vi "provide_OME_data.vi"(6 "image ID":string, 8 "error in (no error)":errorcluster, 9 "structuredAttribute string in":string, 10 "OME element in":refnum<class "XMLElement.lvclass">, 11 "DataCollectionDL091104Scaffold in":refnum<class "DataCollectionDL091104Scaffold.lvclass">) -> (0 "error out":errorcluster, 1 "structuredAttribute string out":string, 2 "OME element out":refnum<class "XMLElement.lvclass">, 3 "DataCollectionDL091104Scaffold out":refnum<class "DataCollectionDL091104Scaffold.lvclass">)   [LabVIEW 2010, in "DataCollectionDL091104Scaffold.lvclass"]
uses:
  DataCollectionDL091104Scaffold.lvclass
  common/classes/XMLElement/XMLElement/XMLElement.lvclass
  GenericDataCollection/GenericDataCollection/GenericDataCollection.lvclass
  DataCollectionDL091104Scaffold.lvclass/DataCollectionDL091104Scaffold.ctl
  Instrument/GenericInstrument/GenericInstrument/GenericInstrument.lvclass
  Objective/GenericObjective/GenericObjective/GenericObjective.lvclass
  common/classes/ErrorController/ErrorController/class_data.vi
  common/classes/ErrorController/ErrorController/ErrorController.lvclass
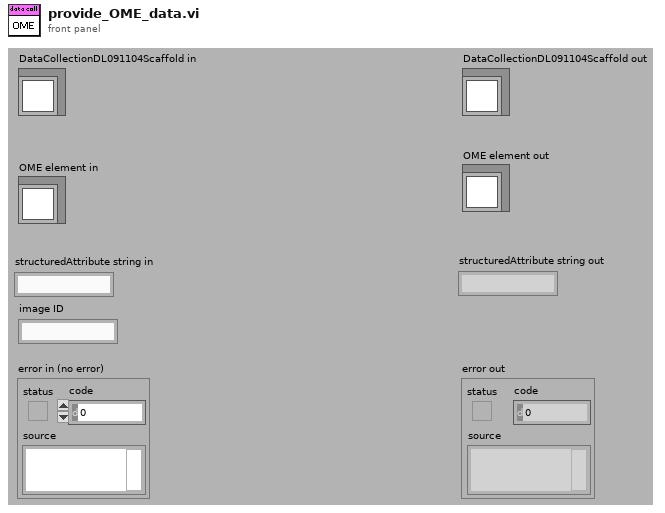
[diagram p1: front panel]
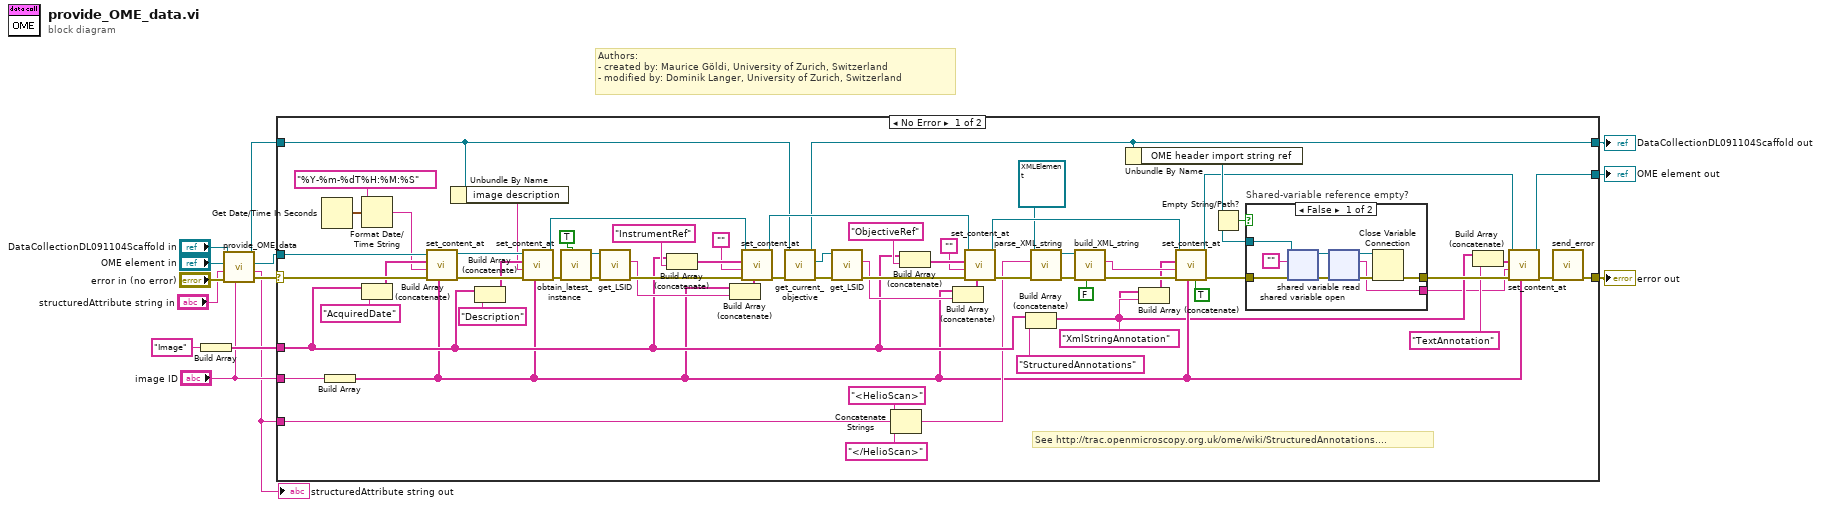
[diagram p0: block diagram]
diagram:
  # "Authors: \n- created by: Maurice Göldi, University of Zurich, Switzerland\n- modified by: Dominik Langer, University of Zurich, Switzerland"
  n1 = Build Array("Image") -> (w10:string[])
  n2 = call-parent "provide_OME_data.vi"("image ID"="image ID", "error in (no error)"="error in (no error)", "structuredAttribute string in"="structuredAttribute string in", "OME element in"="OME element in", "GenericDataCollection in"="DataCollectionDL091104Scaffold in") -> ("error out"=w9:errorcluster, "structuredAttribute string out"=w1:string, "OME element out"=w8:refnum<class "XMLElement.lvclass">, "GenericDataCollection out"=w7:refnum<class "DataCollectionDL091104Scaffold.lvclass">)  [unwired: 3 in]
  "structuredAttribute string out" <- w1
  n3 = case shown="No Error" w9 {
    selector: w9 -> [w71 w93]
    tunnel: [w50 w93] -> w6
    tunnel: w10 -> [w38 _]
    tunnel: "image ID" -> [w75 _]
    tunnel: w8 -> [w69 w91]
    tunnel: w7 -> [w51 w92]
    tunnel: [w49 w92] -> w5
    tunnel: [w21 w91] -> w4
    tunnel: w1 -> [w29 _]
    frame No Error {
      # "See http://trac.openmicroscopy.org.uk/ome/wiki/StructuredAnnotations...."
      n4 = Get Date/Time In Seconds() -> (seconds since 1Jan1904=w74:timestamp)
      n5 = Build Array(w75) -> (w20:string[])
      n6 = Format Date/Time String(time format string (%c)="%Y-%m-%dT%H:%M:%S", seconds (now)=w74) -> (date/time string=w44:string)  [unwired: 1 in]
      n7 = Build Array (concatenate)(w38, "AcquiredDate" ("String")) -> (w70:string[])
      n8 = call "set_content_at.vi"("id chain"=w20, "error in (no error)"=w71, "content"=w44, "key chain"=w70, "Element in"=w69) -> ("error out"=w72:errorcluster, "Element out"=w68:refnum<class "XMLElement.lvclass">)  [unwired: 5 in]
      n9 = Unbundle By Name(w51) -> ("image description"=w43:string)
      n10 = Build Array (concatenate)(w38, "Description" ("String")) -> (w67:string[])
      n11 = call "set_content_at.vi"("id chain"=w20, "error in (no error)"=w72, "content"=w43, "key chain"=w67, "Element in"=w68) -> ("error out"=w62:errorcluster, "Element out"=w65:refnum<class "XMLElement.lvclass">)  [unwired: 5 in]
      n12 = call "obtain_latest_instance.vi"("quick, but maybe outdated?"=TRUE, "error in (no error)"=w62) -> ("error out"=w59:errorcluster, "microscope"=w60:refnum<class "GenericInstrument.lvclass">)  [unwired: 8 in]
      n13 = call-dynamic "get_LSID.vi"("error in (no error)"=w59, "GenericPlugin in"=w60) -> ("error out"=w58:errorcluster, "LSID (string)"=w57:string)  [unwired: 6 in, 2 out]
      n14 = Build Array (concatenate)(w38, "InstrumentRef" ("String")) -> (w66:string[])
      n15 = Build Array (concatenate)(w20, w57) -> (w46:string[])
      n16 = call "set_content_at.vi"("id chain"=w46, "error in (no error)"=w58, "content"="", "key chain"=w66, "Element in"=w65) -> ("error out"=w55:errorcluster, "Element out"=w64:refnum<class "XMLElement.lvclass">)  [unwired: 5 in]
      n17 = call-dynamic "get_current_objective.vi"("error in (no error)"=w55, "GenericPlugin in"=w51) -> ("error out"=w56:errorcluster, "current objective"=w53:refnum<class "GenericObjective.lvclass">, "GenericPlugin out"=w49:refnum<class "DataCollectionDL091104Scaffold.lvclass">)  [unwired: 7 in]
      n18 = call-dynamic "get_LSID.vi"("error in (no error)"=w56, "GenericPlugin in"=w53) -> ("error out"=w54:errorcluster, "LSID (string)"=w52:string)  [unwired: 6 in, 2 out]
      n19 = Concatenate Strings("<HelioScan>" ("string"), w29, "</HelioScan>" ("string")) -> (w30:string)
      n20 = Build Array (concatenate)(w38, "ObjectiveRef" ("String")) -> (w63:string[])
      n21 = Build Array (concatenate)(w20, w52) -> (w45:string[])
      n22 = call "set_content_at.vi"("id chain"=w45, "error in (no error)"=w54, "content"="", "key chain"=w63, "Element in"=w64) -> ("error out"=w35:errorcluster, "Element out"=w40:refnum<class "XMLElement.lvclass">)  [unwired: 5 in]
      n23 = Build Array (concatenate)(w38, "StructuredAnnotations" ("String")) -> (w17:string[])
      n24 = call "parse_XML_string.vi"("error in (no error)"=w35, "XML string"=w30, "Element in"=refnum<class "XMLElement.lvclass"> refnum ("XMLElement.lvclass")) -> ("error out"=w36:errorcluster, "Element out"=w33:refnum<class "XMLElement.lvclass">)  [unwired: 7 in]
      n25 = call "build_XML_string.vi"("pretty print?"=FALSE, "error in (no error)"=w36, "Element in"=w33) -> ("error out"=w34:errorcluster, "string"=w32:string)  [unwired: 6 in, 1 out]
      n26 = Unbundle By Name(w49) -> ("OME header import string ref"=w47:refnum<k21>)
      n27 = Build Array (concatenate)(w17, "XmlStringAnnotation" ("String")) -> (w19:string[])
      n28 = call "set_content_at.vi"("value is XML itself?"=TRUE, "id chain"=w20, "error in (no error)"=w34, "content"=w32, "key chain"=w19, "Element in"=w40) -> ("error out"=w39:errorcluster, "Element out"=w22:refnum<class "XMLElement.lvclass">)  [unwired: 4 in]
      n29 = Empty String/Path?(string/path=w47) -> (empty?=w48:bool)
      n30 = case "Shared-variable reference empty?" shown="False" w48 {
        tunnel: w39 -> [w89 w90]
        tunnel: w47 -> [w88 _]
        tunnel: [w82 _] -> w15
        tunnel: [w81 w90] -> w23
        frame False {
          n31 = shared-variable-open(w88, w89, "") -> (w86:refnum<k21>, w87:errorcluster)  [unwired: 1 in]
          n32 = shared-variable-read(w86, w87) -> (w83:refnum<k21>, w84:errorcluster, w82:string)  [unwired: 1 out]
          n33 = Close Variable Connection(8:w84, 11:w83) -> (0:w81:errorcluster)
        }
        frame True {
        }
      }
      n34 = Build Array (concatenate)(w17, "TextAnnotation" ("String")) -> (w18:string[])
      n35 = call "set_content_at.vi"("id chain"=w20, "error in (no error)"=w23, "content"=w15, "key chain"=w18, "Element in"=w22) -> ("error out"=w24:errorcluster, "Element out"=w21:refnum<class "XMLElement.lvclass">)  [unwired: 5 in]
      n36 = call "send_error.vi"("error in (no error)"=w24) -> ("error out"=w50:errorcluster)  [unwired: 10 in]
    }
    frame Error {
    }
  }
  "error out" <- w6
  "DataCollectionDL091104Scaffold out" <- w5
  "OME element out" <- w4
